vi "Get MessageName.vi"(8 "error in (no error)":errorcluster, 11 "Message in":refnum<class "Message.lvclass">) -> (0 "error out":errorcluster, 2 "Message Name":string, 3 "Message out":refnum<class "Message.lvclass">)   [LabVIEW 2009, in "LapDog.Messaging.v2.lvlib" / "Message.lvclass"]
doc: "Returns the <b>message name</b> (not class name) of the message object on the wire at runtime. The message name can be set when the message object was created or changed using the RenameMessage method. If a message does not have a name, the name of the class (without the file extension) is returned.\n\nThis method executes regardless of the error in state."
uses:
  Message.lvclass
  Message.lvclass/Message.ctl
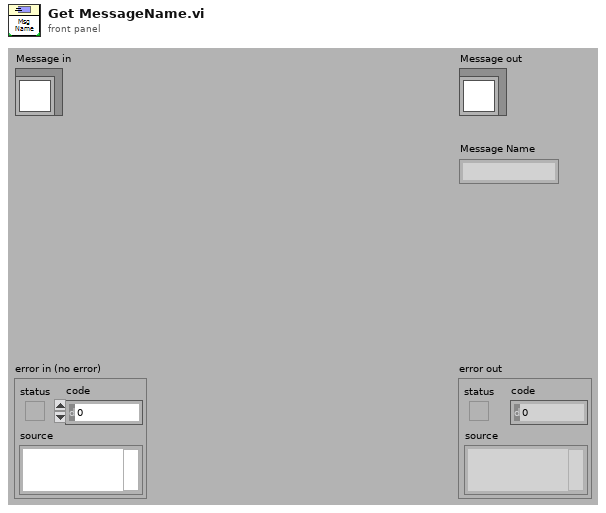
[diagram p1: front panel]
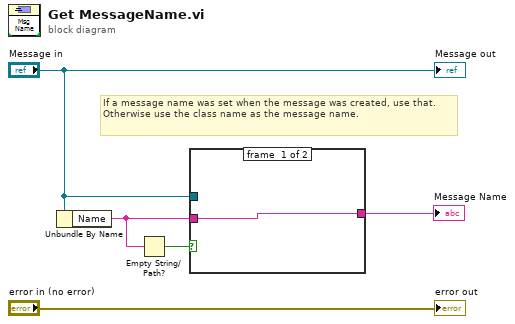
[diagram p0: block diagram]
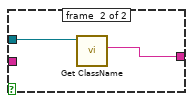
[diagram p2: hidden frame]
diagram:
  # "If a message name was set when the message was created, use that.  Otherwise use the class name as the message name."
  n1 = Unbundle By Name("Message in") -> ("Name"=w1:string)
  n2 = Empty String/Path?(string/path=w1) -> (empty?=w2:bool)
  n3 = case shown="True" w2 {
    tunnel: [w6 w7] -> w5
    tunnel: "Message in" -> [_ w8]
    tunnel: w1 -> [w6 _]
    frame #0 {
    }
    frame #1 {
      n4 = call "Get ClassName.vi"("Message in"=w8) -> ("Class Name"=w7:string)  [unwired: 8 in, 2 out]
    }
  }
  "Message Name" <- w5
  "error out" <- "error in (no error)"
  "Message out" <- "Message in"
